vi "ReadMultipleDigitalOutputs.vi"(8 "error in (no error)":errorcluster, 11 "DigitalOutput_Simulation In":refnum<class "TesteractHAL_DigitalOutput_Simulation.lvclass">) -> (0 "error out":errorcluster, 2 "data":bool[](array[boolean]), 3 "DigitalOutput_Simulation Out":refnum<class "TesteractHAL_DigitalOutput_Simulation.lvclass">)   [LabVIEW 2017, in "TesteractHAL_DigitalOutput_Simulation.lvlib" / "TesteractHAL_DigitalOutput_Simulation.lvclass"]
doc: "Read multiple lines as single boolean points."
uses:
  TesteractHAL_DigitalOutput_Simulation.lvclass
  TesteractHAL_DigitalOutput_Simulation.lvclass/TesteractHAL_DigitalOutput_Simulation.ctl
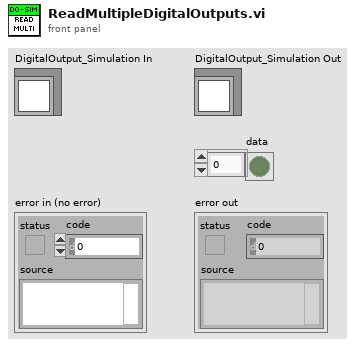
[diagram p1: front panel]
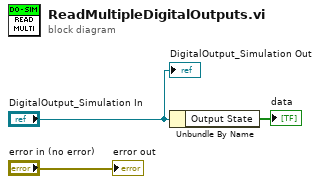
[diagram p0: block diagram]
diagram:
  n1 = Unbundle By Name("DigitalOutput_Simulation In") -> ("Output State"=→"data":bool[])
  "error out" <- "error in (no error)"
  "DigitalOutput_Simulation Out" <- "DigitalOutput_Simulation In"
